vi "Read Model.vi"(8 "error in":errorcluster, 11 "Base Software in":refnum<class "Base Software.lvclass">) -> (0 "error out":errorcluster, 2 "Model":string, 3 "Base Software out":refnum<class "Base Software.lvclass">)   [LabVIEW 2019, in "Base Software.lvlib" / "Main.lvlib" / "Base Software.lvclass"]
uses:
  Project/Base Software.lvclass
  Project/Base Software.lvclass/Base Software.ctl
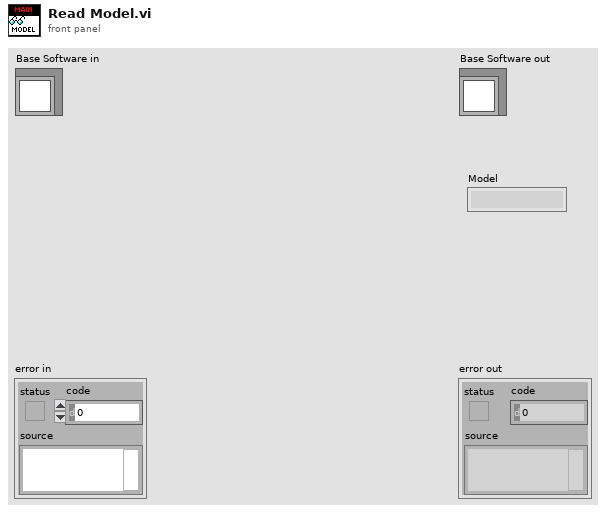
[diagram p1: front panel]
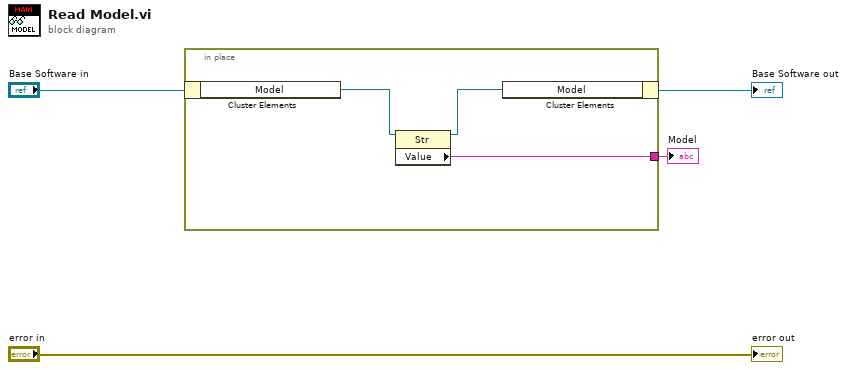
[diagram p0: block diagram]
diagram:
  n1 = in-place {
    in-place-border: [w7] -> w2
    n2 = in-place-cluster #1("Base Software in") -> ("Model"=w6:refnum<vi>)
    n3 = property class="Str"(reference=w6) -> (reference out=w5:refnum<vi>, "Value"=w7:string)  [unwired: 1 in, 1 out]
    n4 = in-place-cluster #1("Model"=w5) -> (→"Base Software out":refnum<class "Base Software.lvclass">)
  }
  "Model" <- w2
  "error out" <- "error in"
